vi "读写串口配置XML.vi"(7 "error in (no error)":errorcluster caption="错误输入（无错误）", 8 "模式":enum16{"Read", "Write"}(ring), 9 "XML File Path":path caption="XML文件路径", 10 "串口配置.lvclass In":refnum<class "串口配置.lvclass">) -> (0 "error out":errorcluster caption="错误输出", 3 "串口配置.Out":refnum<class "串口配置.lvclass">)   [LabVIEW 2013, in "串口配置.lvclass"]
uses:
  <vilib>/Utility/xml.llb/Read From XML File(string).vi
  <vilib>/Utility/xml.llb/Write to XML File(string).vi
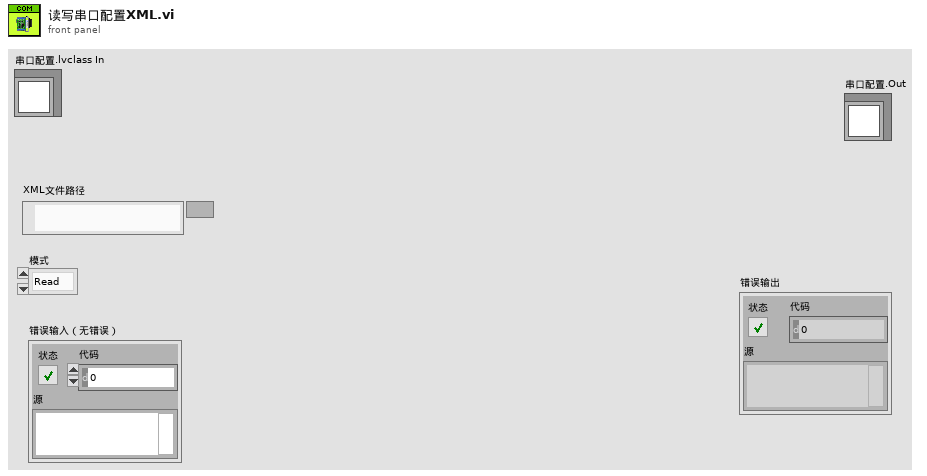
[diagram p1: front panel]
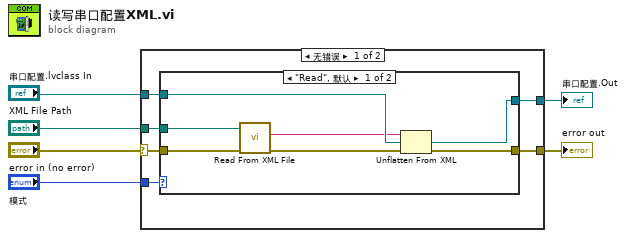
[diagram p0: block diagram]
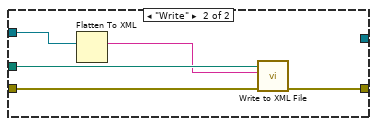
[diagram p2: hidden frame]
diagram:
  n1 = case shown="无错误" "error in (no error)" {
    selector: "error in (no error)" -> [w8 w25]
    tunnel: [w10 w25] -> w5
    tunnel: "XML File Path" -> [w12 _]
    tunnel: "串口配置.lvclass In" -> [w11 _]
    tunnel: [w9 _] -> w2
    tunnel: "模式" -> [w7 _]
    frame No Error {
      n2 = case shown="\"Read\", 默认" w7 {
        tunnel: w12 -> [w19 w23]
        tunnel: w11 -> [w17 w24]
        tunnel: [w15 w20] -> w10
        tunnel: [w14 _] -> w9
        tunnel: w8 -> [w13 w21]
        frame "Read", Default {
          n3 = call-poly <vilib>:"Read From XML File.vi"("error in (no error)"=w13, "XML File Path"=w19) -> ("error out"=w18:errorcluster, "XML Elements"=w16:string)  [unwired: 7 in, 1 out]
          n4 = Unflatten From XML(xml string=w16, type=w17, error in (no error)=w18) -> (value=w14:refnum<class "串口配置.lvclass">, error out=w15:errorcluster)
        }
        frame "Write" {
          n5 = Flatten To XML(anything=w24) -> (xml string=w22:string)
          n6 = call-poly <vilib>:"Write to XML File.vi"("error in (no error)"=w21, "XML Input"=w22, "XML File Path"=w23) -> ("error out"=w20:errorcluster)  [unwired: 6 in, 2 out]
        }
      }
    }
    frame Error {
    }
  }
  "串口配置.Out" <- w2
  "error out" <- w5
